vi "AuthorizationUpdated.vi"(8 "ErrorIn":errorcluster, 11 "ReferenceIn":refnum<class "DemoApplication.lvclass">) -> (0 "ErrorOut":errorcluster, 3 "ReferenceIn":refnum<class "DemoApplication.lvclass">)   [LabVIEW 2021, in "DemoApplication.lvclass"]
uses:
  DemoApplication.lvclass
  .Externals/Interface_TAF_IAuthorization/IAuthorization/IAuthorization.lvclass
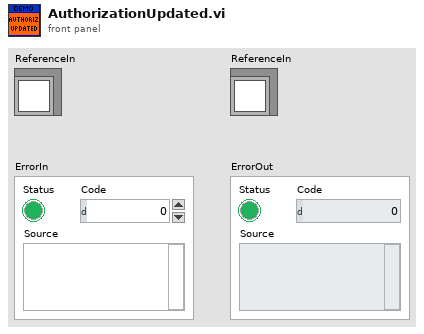
[diagram p1: front panel]
types:
  T1 = typedef "DemoApplication.lvclass/ObjectAttributes.ctl" = cluster{"Interfaces":cluster{"Authorizer":refnum<class "IAuthorization.lvclass">, "TextViewer":refnum<class "ITAFTextViewer.lvclass">, "ApplicationConfiguration":refnum<class "IApplicationConfiguration.lvclass">, "Tracer":refnum<class "IFrontPanel.lvclass">}, "Persistent":cluster{"MenuEnables":cluster{"MenuTag":string, "MenuExpression":string}[], "TextDockSubPanelName":string}}
  T2 = cluster{"MenuTag":string, "MenuExpression":string}[]
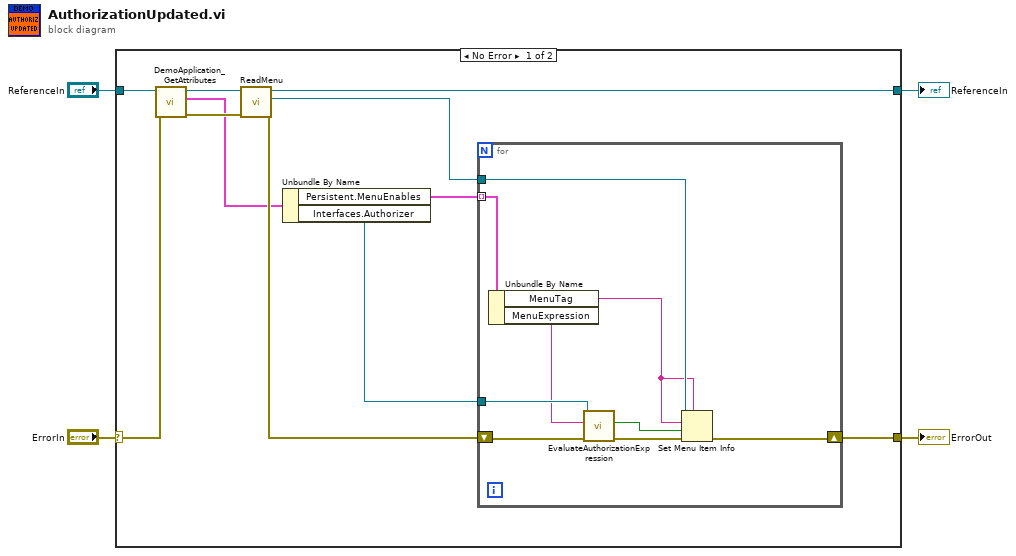
[diagram p0: block diagram]
diagram:
  n1 = case shown="No Error" "ErrorIn" {
    selector: "ErrorIn" -> [w15 w26]
    tunnel: [w14 w26] -> w3
    tunnel: [w6 w25] -> w1
    tunnel: "ReferenceIn" -> [w10 w25]
    frame No Error {
      n2 = call "DemoApplication_GetAttributes.vi"("ErrorIn"=w15, "ReferenceIn"=w10) -> ("ErrorOut"=w13:errorcluster, "Data"=w11:T1, "ReferenceOut"=w7:refnum<class "DemoApplication.lvclass">)  [unwired: 6 in, 1 out]
      n3 = call-dynamic "ReadMenu.vi"("ErrorIn"=w13, "ReferenceIn"=w7) -> ("ErrorOut"=w12:errorcluster, "Menu"=w5:refnum<k9>, "ReferenceIn"=w6:refnum<class "DemoApplication.lvclass">)  [unwired: 7 in]
      n4 = Unbundle By Name(w11) -> ("Persistent.MenuEnables"=w9:T2, "Interfaces.Authorizer"=w8:refnum<class "IAuthorization.lvclass">)
      n5 = for {
        tunnel: w9 -> [w20] mode=indexing
        shift-right: [w22] -> w14
        shift-left: w12 -> [w24]
        tunnel: w8 -> [w21]
        tunnel: w5 -> [w18]
        n6 = Unbundle By Name(w20) -> ("MenuTag"=w16:string, "MenuExpression"=w19:string)
        n7 = call-dynamic "EvaluateAuthorizationExpression.vi"("ErrorIn"=w24, "Expression"=w19, "ReferenceIn"=w21) -> ("ErrorOut"=w23:errorcluster, "Pass"=w17:bool)  [unwired: 5 in, 2 out]
        n8 = Set Menu Item Info(7:w16, 8:w23, 9:w17, 10:w16, 11:w18) -> (0:w22:errorcluster)  [unwired: 2 in, 1 out]
      }
    }
    frame Error {
    }
  }
  "ErrorOut" <- w3
  "ReferenceIn" <- w1
